vi "lua_typename.vi"(8 "error in (no error)":errorcluster, 10 "lua type":T1 items=["LUA_TNONE"=-1, "LUA_TNIL"=0, "LUA_TBOOLEAN"=1, "LUA_TLIGHTUSERDATA"=2, "LUA_TNUMBER"=3, "LUA_TSTRING"=4, "LUA_TTABLE"=5, "LUA_TFUNCTION"=6, "LUA_TUSERDATA"=7, "LUA_TTHREAD"=8, "LUA_NUMTYPES"=9], 11 "lua_state_p in":u64) -> (0 "error out":errorcluster, 2 "lua_state_p":u64, 3 "result":string)   [LabVIEW 2020, in "lua.dll.lvlib"]
uses:
  lua.dll.lvlib
  lua_types.ctl
  lua54.dll
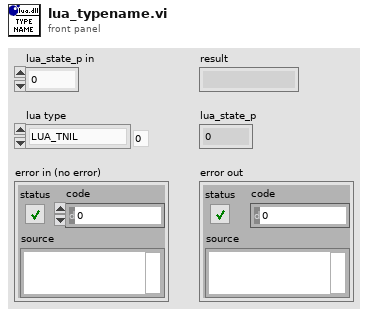
[diagram p1: front panel]
types:
  T1 = typedef "lua.dll.lvlib/lua_types.ctl" = i32
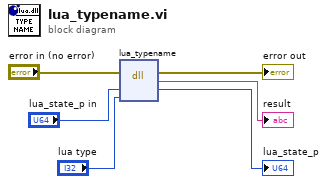
[diagram p0: block diagram]
diagram:
  n1 = dll-call lib="C:/Users/Nicholas Folse/Documents/workspace/github-tauterra.llc/Lua for LabVIEW/lib/lua.dll/lua54**.*" fn="lua_typename"(error in="error in (no error)", "lua_state_p"="lua_state_p in", "type"="lua type") -> (error out=→"error out":errorcluster, "result"=→"result":string, "lua_state_p"=→"lua_state_p":u64)  [unwired: 3 in, 1 out]
